vi "Get Phase Temperature Coefficients.vi"(0 "VISA resource name":refnum<visa-resource-name>, 5 "ACM Path":T2, 7 "S-Parameter":T1, 11 "error in (no error)":errorcluster) -> (4 "VISA resource name out":refnum<visa-resource-name>, 8 "Phase Coefficients":dbl[](array[numeric]), 15 "error out":errorcluster)   [LabVIEW 2023, in "ACM Visa Driver.lvlib"]
uses:
  ACM Visa Driver.lvlib
  Controls/ACM Paths.ctl
  Controls/ACM S-Parameters.ctl
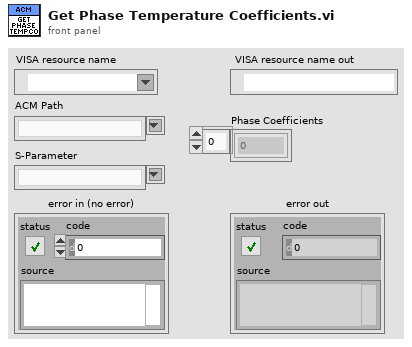
[diagram p1: front panel]
types:
  T1 = typedef "ACM Visa Driver.lvlib/ACM S-Parameters.ctl" = string
  T2 = typedef "ACM Visa Driver.lvlib/ACM Paths.ctl" = string
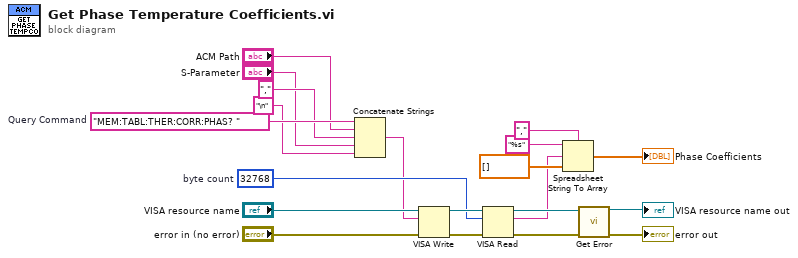
[diagram p0: block diagram]
diagram:
  w11 = "MEM:TABL:THER:CORR:PHAS? "  # Query Command
  w15 = u32 32768  # byte count
  n1 = Concatenate Strings(w11, "ACM Path", ",", "S-Parameter", "\n") -> (w6:string)
  n2 = VISA Write(VISA resource name="VISA resource name", write buffer=w6, error in (no error)="error in (no error)") -> (VISA resource name out=w16:refnum<visa-resource-name>, error out=w18:errorcluster)  [unwired: 1 out]
  n3 = VISA Read(VISA resource name=w16, byte count=w15, error in (no error)=w18) -> (VISA resource name out=w13:refnum<visa-resource-name>, read buffer=w2:string, error out=w17:errorcluster)  [unwired: 1 out]
  n4 = Spreadsheet String To Array(delimiter (Tab)=",", format string="%s", spreadsheet string=w2, array type (2D Dbl)=dbl[] []) -> (array=→"Phase Coefficients":dbl[])
  n5 = call "Get Error.vi"("VISA resource name"=w13, "error in (no error)"=w17) -> ("VISA resource name out"=→"VISA resource name out":refnum<visa-resource-name>, "error out"=→"error out":errorcluster)  [unwired: 12 in]
